vi "p8.1.vi"() -> ()   [LabVIEW 2020]
panel:
  out "File Data Type out":i32
  out "File Type out":string
  out "error out":errorcluster
  out "Image":T1(plugin-control)
  in  "File Path":path
  in  "Image Type":T2 items=["Grayscale (U8)", "Grayscale (I16)", "Grayscale (SGL)", "Complex (CSG)", "RGB (U32)", "HSL (U32)", "RGB (U64)", "Grayscale (U16)"]
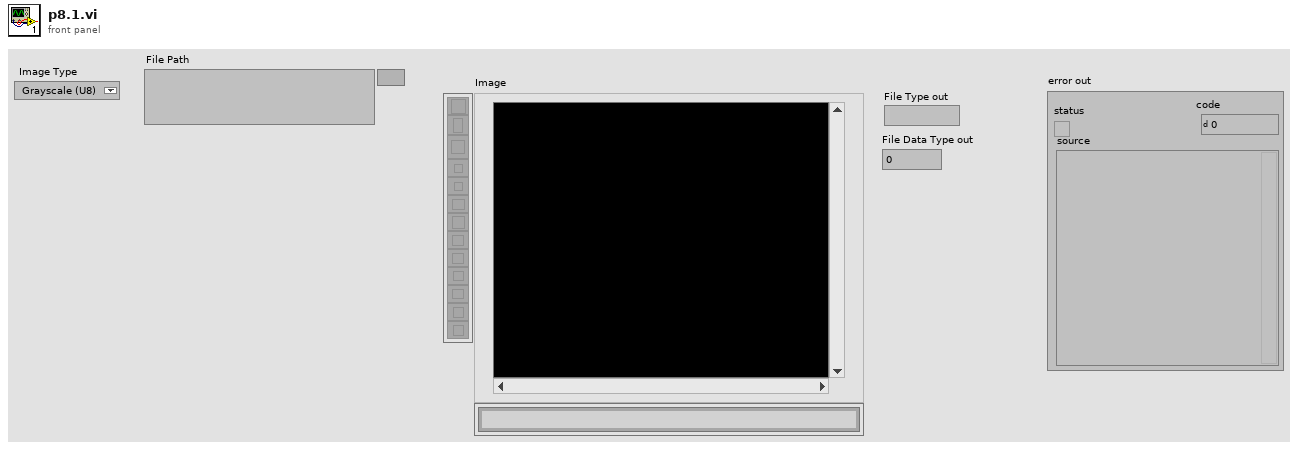
[diagram p1: front panel]
types:
  T1 = typedef "IMAQ Image.ctl" = refnum<image>
  T2 = typedef "Image Type" = u32
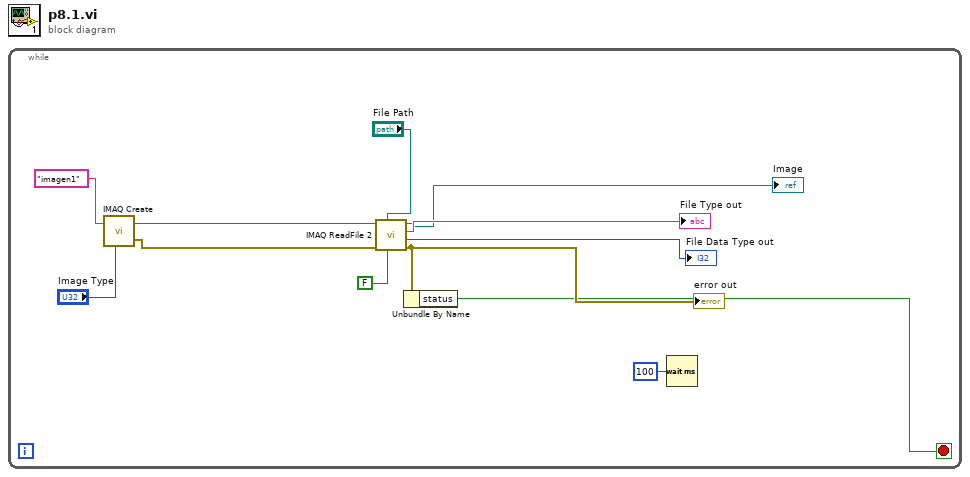
[diagram p0: block diagram]
diagram:
  n1 = while {
    stop <- w4 stop-if-true
    n2 = call "IMAQ Create"("Image Name"="imagen1", "Image Type"="Image Type") -> ("New Image"=w12:T1, "error out"=w11:errorcluster)  [unwired: 3 in]
    n3 = call "IMAQ ReadFile 2"("Use File Path Image Type"=FALSE, "File Path"="File Path", "error in (no error)"=w11, "Image"=w12) -> ("error out"=w5:errorcluster, "File Data Type out"=→"File Data Type out":i32, "File Type out"=→"File Type out":string, "Image Out"=→"Image":T1)  [unwired: 3 in, 1 out]
    "error out" <- w5
    n4 = Unbundle By Name(w5) -> ("status"=w4:bool)
    n5 = Wait (ms)(milliseconds to wait=u32 100) -> ()  [unwired: 1 out]
  }
